vi "read_VDCInputErrors2.vi"(1 "Array":u8[](array[numeric])=[0, 0, 0, 0, 0, 0, 0, 0, 0, 0, 0, 0, 0, 0, 0, 0, 0, 0, 0, 0, 0, 0, 0, 0, 0, 0, 0, 0, 0, 0, 0, 0, 0, 0, 0, 0, 0, 0, 0, 0, 0, 0, 0, 0, 0, 0, 0, 0, 0, 0, 0, 0, 0, 0, 0, 0, 0, 0, 0, 0, 0, 0, 0, 0, 0, 0, 0, 0, 0, 0, 0, 0, 0, 0, 0, 0, 0, 0, 0, 0, 0, 0, 0, 0, 0, 0, 0, 0, 0, 0, 0, 0, 0, 0, 0, 0, 0, 0, 0, 0, 0, 0, 0, 0, 0, 0, 0, 0, 0, 0, 0, 0, 0, 0, 0, 0, 0, 0, 0, 0, 0, 0, 0, 0, 0, 0, 0, 0, 0, 0, 0, 0, 0, 0, 0, 0, 0, 0, 0, 0, 0, 0, 0, 0, 0, 0, 0, 0, 0, 0, 0, 0, 0, 0, 0, 0, 0, 0, 0, 0, 0, 0, 0, 0, 0, 0, 0, 0, 0, 0, 0, 0, 0, 0, 0, 0, 0, 0, 0, 0, 0]) -> (0 "output cluster":T1)   [LabVIEW 2017]
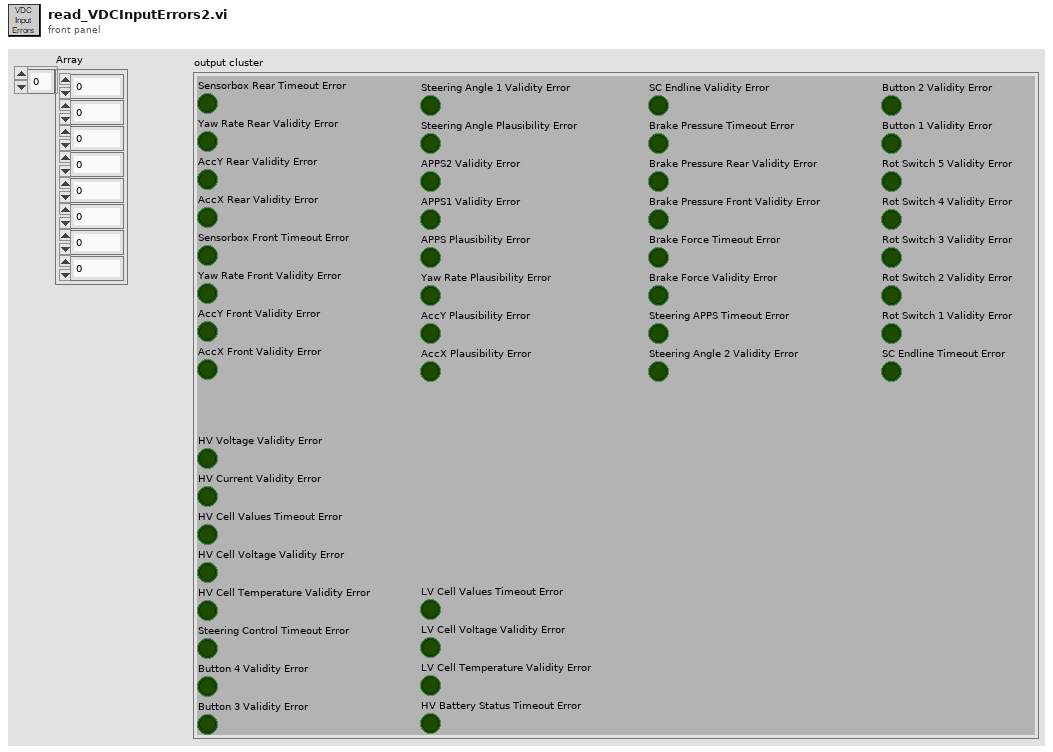
[diagram p1: front panel]
types:
  T1 = cluster{"Sensorbox Rear Timeout Error ":bool, "Yaw Rate Rear Validity Error ":bool, "AccY Rear Validity Error":bool, "AccX Rear Validity Error ":bool, "Sensorbox Front Timeout Error":bool, "Yaw Rate Front Validity Error":bool, "AccY Front Validity Error":bool, "AccX Front Validity Error":bool, "Steering Angle 1 Validity Error":bool, "Steering Angle Plausibility Error":bool, "APPS2 Validity Error":bool, "APPS1 Validity Error":bool, "APPS Plausibility Error ":bool, "Yaw Rate Plausibility Error ":bool, "AccY Plausibility Error ":bool, "AccX Plausibility Error ":bool, "SC Endline Validity Error":bool, "Brake Pressure Timeout Error ":bool, "Brake Pressure Rear Validity Error":bool, "Brake Pressure Front Validity Error":bool, "Brake Force Timeout Error ":bool, "Brake Force Validity Error ":bool, "Steering APPS Timeout Error":bool, "Steering Angle 2 Validity Error":bool, "Button 2 Validity Error":bool, "Button 1 Validity Error":bool, "Rot Switch 5 Validity Error":bool, "Rot Switch 4 Validity Error":bool, "Rot Switch 3 Validity Error":bool, "Rot Switch 2 Validity Error":bool, "Rot Switch 1 Validity Error":bool, "SC Endline Timeout Error":bool, "HV Voltage Validity Error":bool, "HV Current Validity Error":bool, "HV Cell Values Timeout Error":bool, "HV Cell Voltage Validity Error":bool, "HV Cell Temperature Validity Error":bool, "Steering Control Timeout Error":bool, "Button 4 Validity Error":bool, "Button 3 Validity Error":bool, "LV Cell Values Timeout Error":bool, "LV Cell Voltage Validity Error":bool, "LV Cell Temperature Validity Error":bool, "HV Battery Status Timeout Error":bool}
  T2 = cluster{"Sensorbox Rear Timeout Error ":bool, "Yaw Rate Rear Validity Error ":bool, "AccY Rear Validity Error":bool, "AccX Rear Validity Error ":bool, "Sensorbox Front Timeout Error  2":bool, "Yaw Rate Front Validity Error":bool, "AccY Front Validity Error":bool, "AccX Front Validity Error":bool, "Steering Angle 1 Validity Error":bool, "Steering Angle Plausibility Error":bool, "APPS2 Validity Error":bool, "APPS1 Validity Error":bool, "APPS Plausibility Error ":bool, "Yaw Rate Plausibility Error ":bool, "AccY Plausibility Error ":bool, "AccX Plausibility Error ":bool, "SC Endline Validity Error":bool, "Brake Pressure Timeout Error ":bool, "Brake Pressure Rear Validity Error":bool, "Brake Pressure Front Validity Error":bool, "Brake Force Timeout Error ":bool, "Brake Force Validity Error ":bool, "Steering APPS Timeout Error":bool, "Steering Angle 2 Validity Error":bool, "Button 2 Validity Error":bool, "Button 1 Validity Error":bool, "Rot Switch 5 Validity Error":bool, "Rot Switch 4 Validity Error":bool, "Rot Switch 3 Validity Error":bool, "Rot Switch 2 Validity Error":bool, "Rot Switch 1 Validity Error":bool, "SC Endline Timeout Error":bool, "HV Voltage Validity Error":bool, "HV Current Validity Error":bool, "HV Cell Values Timeout Error":bool, "HV Cell Voltage Validity Error":bool, "HV Cell Temperature Validity Error":bool, "Steering Control Timeout Error":bool, "Button 4 Validity Error":bool, "Button 3 Validity Error":bool, "LV Cell Values Timeout Error":bool, "LV Cell Voltage Validity Error":bool, "LV Cell Temperature Validity Error":bool, "HV Battery Status Timeout Error":bool}
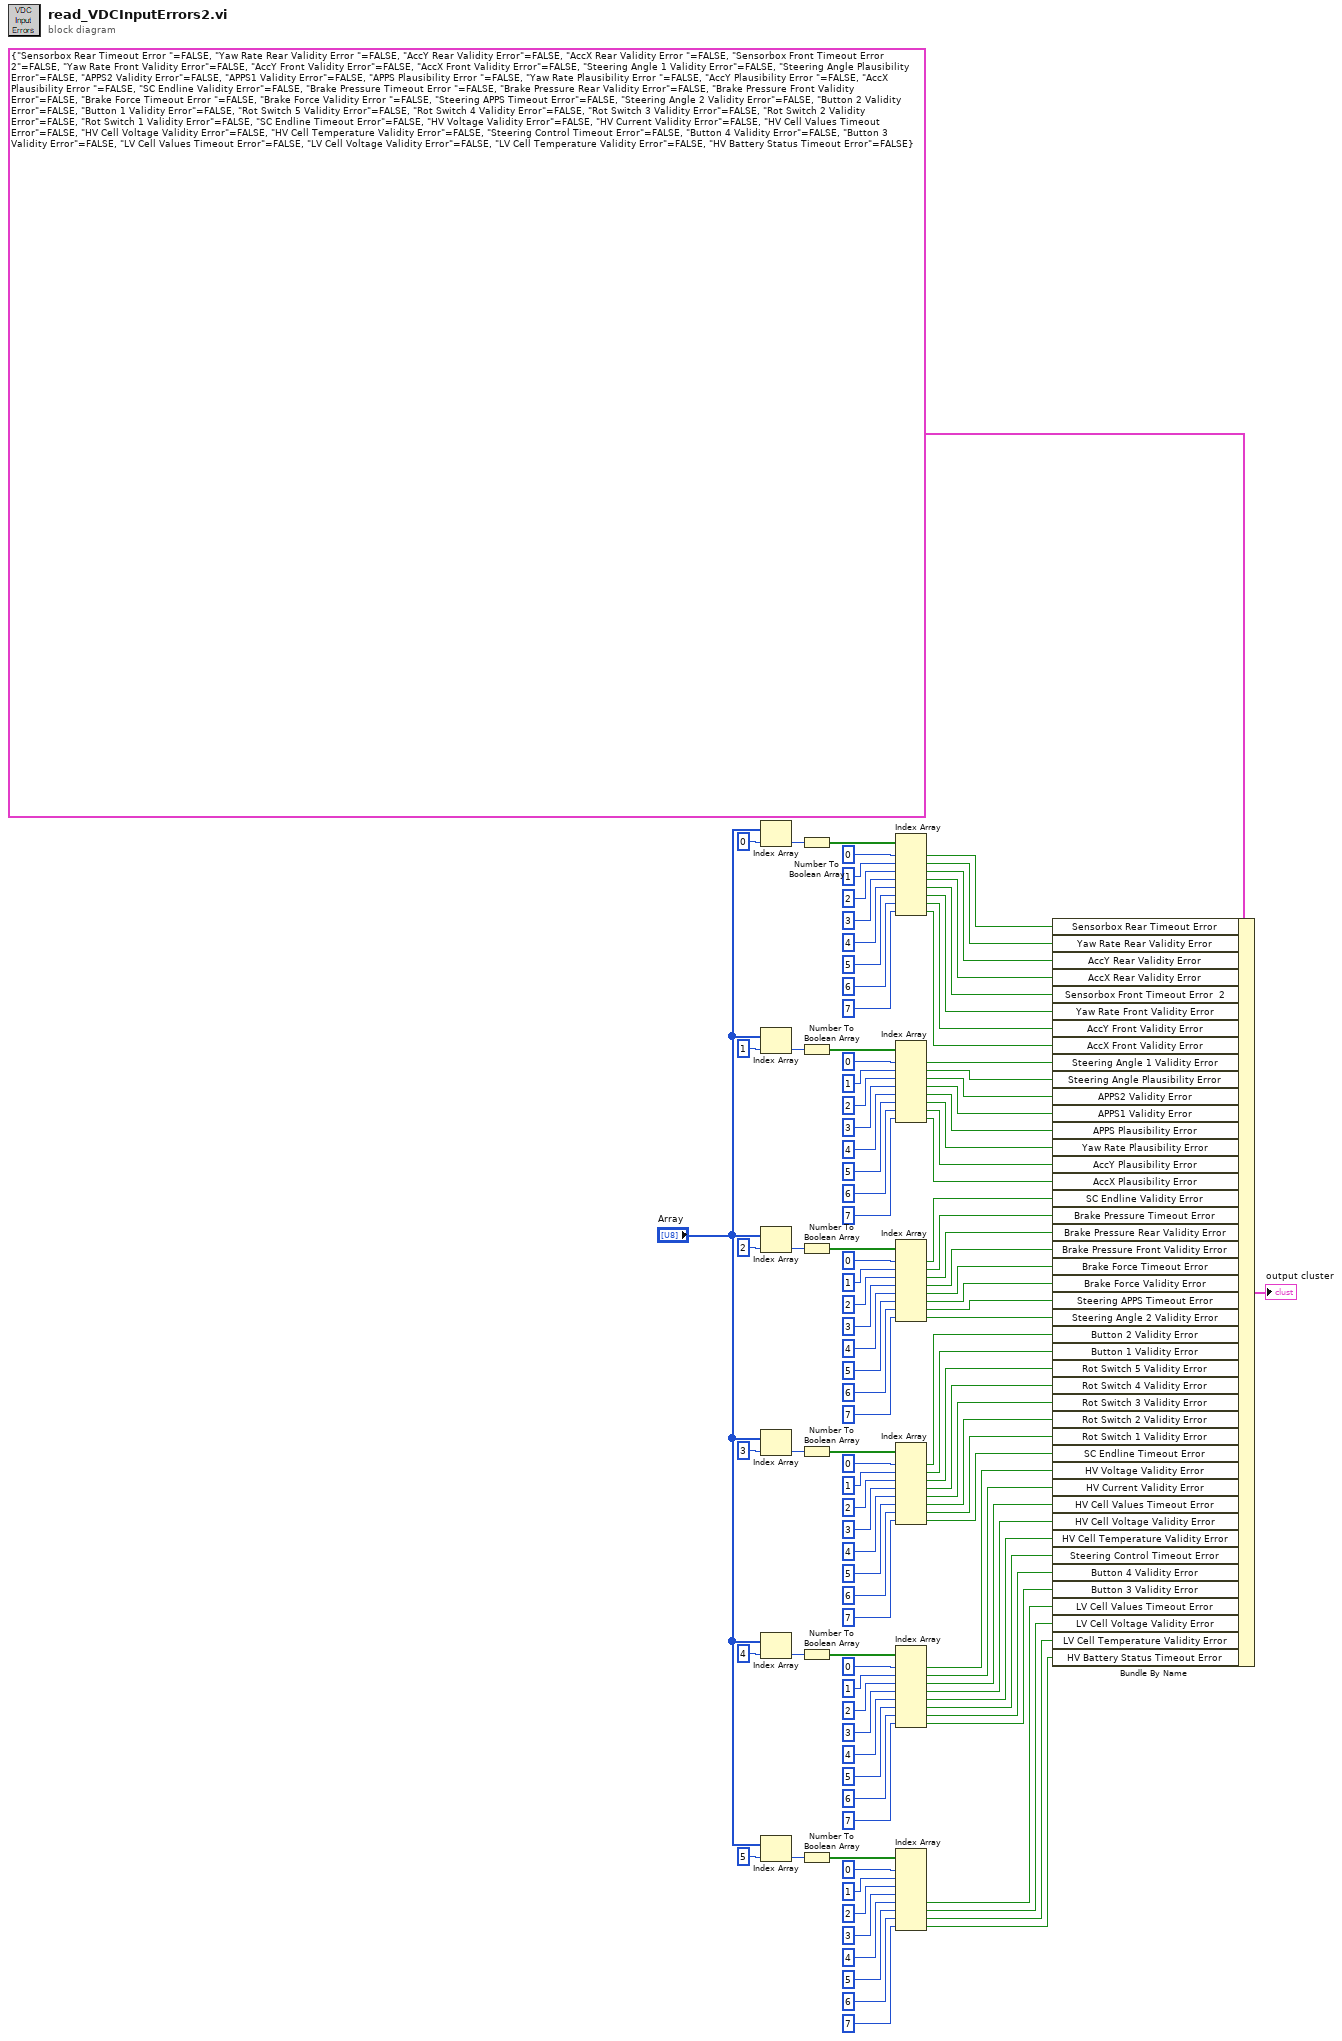
[diagram p0: block diagram]
diagram:
  n1 = Index Array(array="Array", index=0) -> (element=w81:u8)
  n2 = Index Array(array="Array", index=1) -> (element=w102:u8)
  n3 = Index Array(array="Array", index=2) -> (element=w103:u8)
  n4 = Index Array(array="Array", index=3) -> (element=w80:u8)
  n5 = Index Array(array="Array", index=4) -> (element=w61:u8)
  n6 = Index Array(array="Array", index=5) -> (element=w57:u8)
  n7 = Number To Boolean Array(number=w81) -> (Boolean array=w90:bool[])
  n8 = Number To Boolean Array(number=w102) -> (Boolean array=w93:bool[])
  n9 = Number To Boolean Array(number=w103) -> (Boolean array=w112:bool[])
  n10 = Number To Boolean Array(number=w80) -> (Boolean array=w71:bool[])
  n11 = Number To Boolean Array(number=w61) -> (Boolean array=w70:bool[])
  n12 = Number To Boolean Array(number=w57) -> (Boolean array=w48:bool[])
  n13 = Index Array(array=w90, index #1=0 ("index"), index #2=1 ("index"), index #3=2 ("index"), index #4=3 ("index"), index #5=4 ("index"), index #6=5 ("index"), index #7=6 ("index"), index #8=7 ("index")) -> (element #1=w1:bool, element #2=w45:bool, element #3=w44:bool, element #4=w43:bool, element #5=w42:bool, element #6=w41:bool, element #7=w40:bool, element #8=w39:bool)
  n14 = Index Array(array=w93, index #1=0 ("index"), index #2=1 ("index"), index #3=2 ("index"), index #4=3 ("index"), index #5=4 ("index"), index #6=5 ("index"), index #7=6 ("index"), index #8=7 ("index")) -> (element #1=w38:bool, element #2=w37:bool, element #3=w36:bool, element #4=w35:bool, element #5=w34:bool, element #6=w33:bool, element #7=w32:bool, element #8=w31:bool)
  n15 = Index Array(array=w112, index #1=0 ("index"), index #2=1 ("index"), index #3=2 ("index"), index #4=3 ("index"), index #5=4 ("index"), index #6=5 ("index"), index #7=6 ("index"), index #8=7 ("index")) -> (element #1=w30:bool, element #2=w29:bool, element #3=w28:bool, element #4=w27:bool, element #5=w26:bool, element #6=w25:bool, element #7=w24:bool, element #8=w23:bool)
  n16 = Index Array(array=w71, index #1=0 ("index"), index #2=1 ("index"), index #3=2 ("index"), index #4=3 ("index"), index #5=4 ("index"), index #6=5 ("index"), index #7=6 ("index"), index #8=7 ("index")) -> (element #1=w22:bool, element #2=w21:bool, element #3=w20:bool, element #4=w19:bool, element #5=w18:bool, element #6=w17:bool, element #7=w16:bool, element #8=w15:bool)
  n17 = Index Array(array=w70, index #1=0 ("index"), index #2=1 ("index"), index #3=2 ("index"), index #4=3 ("index"), index #5=4 ("index"), index #6=5 ("index"), index #7=6 ("index"), index #8=7 ("index")) -> (element #1=w14:bool, element #2=w13:bool, element #3=w12:bool, element #4=w11:bool, element #5=w10:bool, element #6=w9:bool, element #7=w8:bool, element #8=w7:bool)
  n18 = Index Array(array=w48, index #1=0 ("index"), index #2=1 ("index"), index #3=2 ("index"), index #4=3 ("index"), index #5=4 ("index"), index #6=5 ("index"), index #7=6 ("index"), index #8=7 ("index")) -> (element #5=w6:bool, element #6=w5:bool, element #7=w4:bool, element #8=w3:bool)  [unwired: 4 out]
  n19 = Bundle By Name(cluster=T2 {"Sensorbox Rear Timeout Error "=FALSE, "Yaw Rate Rear Validity Error "=FALSE, "AccY Rear Validity Error"=FALSE, "AccX Rear Validity Error "=FALSE, "Sensorbox Front Timeout Error  2"=FALSE, "Yaw Rate Front Validity Error"=FALSE, "AccY Front Validity Error"=FALSE, "AccX Front Validity Error"=FALSE, "Steering Angle 1 Validity Error"=FALSE, "Steering Angle Plausibility Error"=FALSE, "APPS2 Validity Error"=FALSE, "APPS1 Validity Error"=FALSE, "APPS Plausibility Error "=FALSE, "Yaw Rate Plausibility Error "=FALSE, "AccY Plausibility Error "=FALSE, "AccX Plausibility Error "=FALSE, "SC Endline Validity Error"=FALSE, "Brake Pressure Timeout Error "=FALSE, "Brake Pressure Rear Validity Error"=FALSE, "Brake Pressure Front Validity Error"=FALSE, "Brake Force Timeout Error "=FALSE, "Brake Force Validity Error "=FALSE, "Steering APPS Timeout Error"=FALSE, "Steering Angle 2 Validity Error"=FALSE, "Button 2 Validity Error"=FALSE, "Button 1 Validity Error"=FALSE, "Rot Switch 5 Validity Error"=FALSE, "Rot Switch 4 Validity Error"=FALSE, "Rot Switch 3 Validity Error"=FALSE, "Rot Switch 2 Validity Error"=FALSE, "Rot Switch 1 Validity Error"=FALSE, "SC Endline Timeout Error"=FALSE, "HV Voltage Validity Error"=FALSE, "HV Current Validity Error"=FALSE, "HV Cell Values Timeout Error"=FALSE, "HV Cell Voltage Validity Error"=FALSE, "HV Cell Temperature Validity Error"=FALSE, "Steering Control Timeout Error"=FALSE, "Button 4 Validity Error"=FALSE, "Button 3 Validity Error"=FALSE, "LV Cell Values Timeout Error"=FALSE, "LV Cell Voltage Validity Error"=FALSE, "LV Cell Temperature Validity Error"=FALSE, "HV Battery Status Timeout Error"=FALSE}, "Sensorbox Rear Timeout Error"=w1, "Yaw Rate Rear Validity Error"=w45, "AccY Rear Validity Error"=w44, "AccX Rear Validity Error"=w43, "Sensorbox Front Timeout Error  2"=w42, "Yaw Rate Front Validity Error"=w41, "AccY Front Validity Error"=w40, "AccX Front Validity Error"=w39, "Steering Angle 1 Validity Error"=w38, "Steering Angle Plausibility Error"=w37, "APPS2 Validity Error"=w36, "APPS1 Validity Error"=w35, "APPS Plausibility Error"=w34, "Yaw Rate Plausibility Error"=w33, "AccY Plausibility Error"=w32, "AccX Plausibility Error"=w31, "SC Endline Validity Error"=w30, "Brake Pressure Timeout Error"=w29, "Brake Pressure Rear Validity Error"=w28, "Brake Pressure Front Validity Error"=w27, "Brake Force Timeout Error"=w26, "Brake Force Validity Error"=w25, "Steering APPS Timeout Error"=w24, "Steering Angle 2 Validity Error"=w23, "Button 2 Validity Error"=w22, "Button 1 Validity Error"=w21, "Rot Switch 5 Validity Error"=w20, "Rot Switch 4 Validity Error"=w19, "Rot Switch 3 Validity Error"=w18, "Rot Switch 2 Validity Error"=w17, "Rot Switch 1 Validity Error"=w16, "SC Endline Timeout Error"=w15, "HV Voltage Validity Error"=w14, "HV Current Validity Error"=w13, "HV Cell Values Timeout Error"=w12, "HV Cell Voltage Validity Error"=w11, "HV Cell Temperature Validity Error"=w10, "Steering Control Timeout Error"=w9, "Button 4 Validity Error"=w8, "Button 3 Validity Error"=w7, "LV Cell Values Timeout Error"=w6, "LV Cell Voltage Validity Error"=w5, "LV Cell Temperature Validity Error"=w4, "HV Battery Status Timeout Error"=w3) -> (→"output cluster":T2)
